vi "update_features.vi"(0 "Device In":T1, 5 "Features":string, 11 "Error in":errorcluster) -> (4 "Device Out":T1, 6 "Comm":T2, 15 "Error Out":errorcluster)   [LabVIEW 2019]
uses:
  <userlib>/IoT Devices/_subVIs/HTTPComm.ctl
  Cluster.ctl
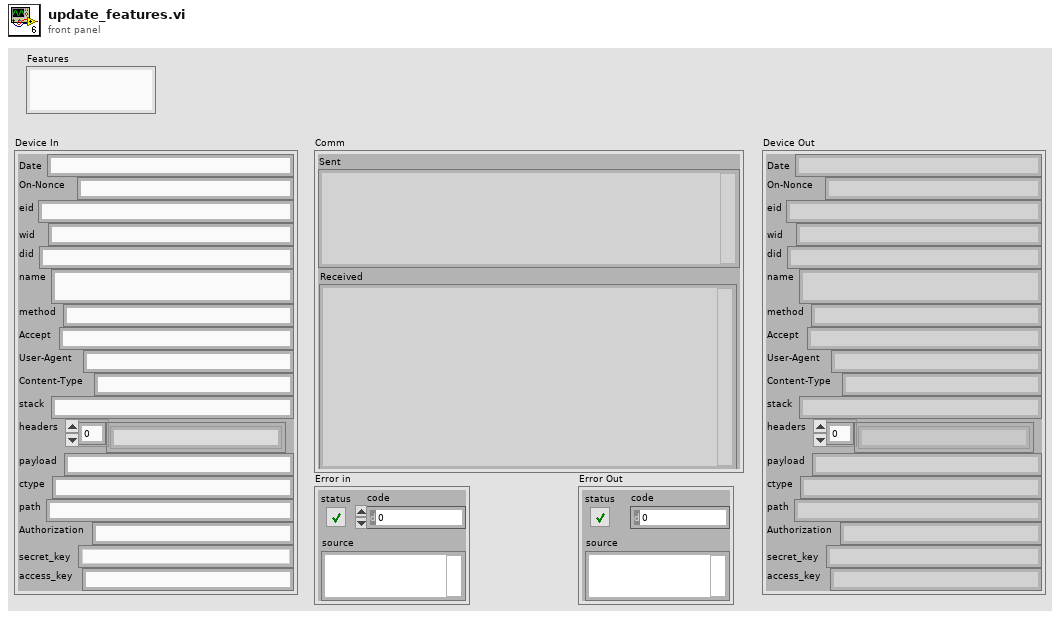
[diagram p1: front panel]
types:
  T1 = typedef "Cluster.ctl" = cluster{"Date":string, "On-Nonce":string, "eid":string, "wid":string, "did":string, "name":string, "method":string, "Accept":string, "User-Agent":string, "Content-Type":string, "stack":string, "headers":string[], "payload":string, "ctype":string, "path":string, "Authorization":string, "secret_key":string, "access_key":string}
  T2 = typedef "HTTPComm.ctl" = cluster{"url":string, "sent headers":string, "sent body":string, "headers":string, "body":string, "Sent":string, "Received":string}
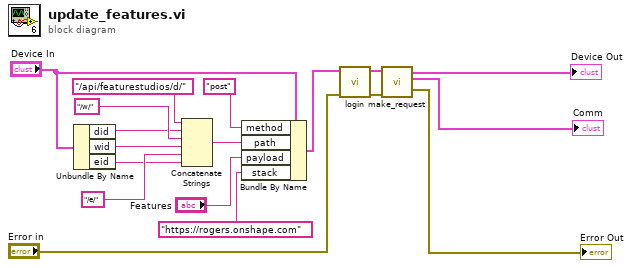
[diagram p0: block diagram]
diagram:
  n1 = Unbundle By Name("Device In") -> ("did"=w7:string, "wid"=w6:string, "eid"=w5:string)
  n2 = Concatenate Strings("/api/featurestudios/d/" ("payload"), w7, "/w/" ("string"), w6, "/e/" ("string"), w5) -> (w14:string)
  n3 = Bundle By Name(cluster="Device In", "method"="post" ("Method"), "path"=w14, "payload"="Features", "stack"="https://rogers.onshape.com" ("stacks")) -> (w8:T1)
  n4 = call "login.vi"("error in"="Error in", "Device In"=w8) -> ("error out"=w10:errorcluster, "Device Out"=w11:T1)  [unwired: 8 in]
  n5 = call "make_request.vi"("Error in"=w10, "Device In"=w11) -> ("error out"=→"Error Out":errorcluster, "Comm"=→"Comm":T2, "Device Out"=→"Device Out":T1)  [unwired: 7 in]
